vi "OpenTalonDrive (3).vi"   [LabVIEW 2016]
uses:
  <vilib>/Rock Robotics/WPI/ThirdParty/CanMotor/TalonSRX/WPI_CANTalonSRX_APIControlMode.ctl
  <vilib>/Rock Robotics/WPI/SafetyOutput/WPI_SafetyOutputConfigMenu.ctl
  <vilib>/Rock Robotics/WPI/ThirdParty/CanMotor/TalonSRX/WPI_CANTalonSRX_APIFeedbackSelect.ctl
types:
  T1 = typedef "WPI_CANTalonSRX_APIFeedbackSelect.ctl" = enum16{"Digital Quadrature Encoder", "Analog Potentiometer", "Analog Encoder", "Count on Quad-A (Rising-Edge)", "Count on Quad-A (Falling-Edge)", "CTR Magnetic Enc (Absolute)", "CTR Magnetic Enc (Relative)", "Pulse Width"}
  T2 = typedef "WPI_SafetyOutputConfigMenu.ctl" = enum16{"Enable", "Disable"}
  T3 = typedef "WPI_CANTalonSRX_APIControlMode.ctl" = enum8{"Percent VBus", "Speed", "Position", "Slave", "Unchanged / Invalid", "Voltage Compensation", "Current", "Motion Profile", "Motion Magic"}
  T4 = typedef "WPI_MotorControlDeviceRef.ctl" = cluster{"DeviceStatus":errorcluster, "Type":T5, "PWM":cluster{"PWM Channel":T6, "DeadBand":T7}, "CAN":cluster{"Device Number":u8, "SetOutput VI Ref":variant, "GetOutput VI Ref":variant, "Enable VI Ref":variant, "Disable VI Ref":variant, "Data":variant}, "Invert":bool}
  T5 = typedef "WPI_MotorControlType.ctl" = enum16{"PWM", "CAN"}
  T6 = typedef "FPGA_DIOPWMChannel.ctl" = enum8{"PWM 0", "PWM 1", "PWM 2", "PWM 3", "PWM 4", "PWM 5", "PWM 6", "PWM 7", "PWM 8", "PWM 9", "PWM MXP 0", "PWM MXP 1", "PWM MXP 2", "PWM MXP 3", "PWM MXP 4", "PWM MXP 5", "PWM MXP 6", "PWM MXP 7", "PWM MXP 8", "PWM MXP 9", "Invalid"}
  T7 = typedef "WPI_PWMDeadband.ctl" = cluster{"Name":string, "maxPositivePwm":i32, "minPositivePwm":i32, "centerPwm":i32, "maxNegativePwm":i32, "minNegativePwm":i32, "angularRange":u16}
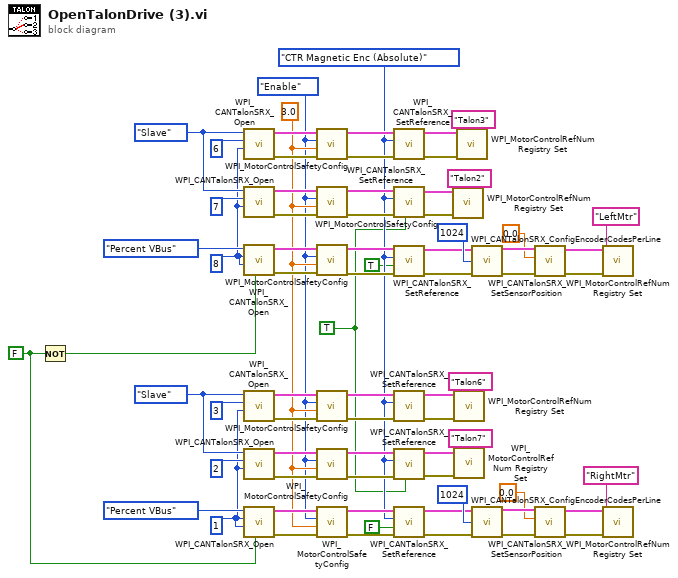
[diagram p0: block diagram]
diagram:
  w4 = FALSE
  w5 = TRUE
  w20 = WPI_CANTalonSRX_APIFeedbackSelect."CTR Magnetic Enc (Absolute)" ("Feedback Reference")
  w37 = WPI_SafetyOutputConfigMenu."Enable" ("mode")
  w7 = u8 1 ("Device Number")
  w55 = WPI_CANTalonSRX_APIControlMode."Slave" ("Control Mode")
  w38 = 3.0 ("timeout (s)")
  w6 = u8 8 ("Device Number")
  w72 = WPI_CANTalonSRX_APIControlMode."Slave" ("Control Mode")
  n1 = Not(x=w4) -> (.not. x?=w3:bool)
  n2 = call <vilib>:"WPI_CANTalonSRX_Open.vi"("Master Device Number"=w6, "Device Number"=u8 6, "Control Mode"=w72) -> ("error out"=w65:errorcluster, "CAN Talon SRX Ref"=w66:T4)  [unwired: 7 in]
  n3 = call <vilib>:"WPI_CANTalonSRX_Open.vi"("Master Device Number"=w6, "Device Number"=u8 7, "Control Mode"=w72) -> ("error out"=w63:errorcluster, "CAN Talon SRX Ref"=w64:T4)  [unwired: 7 in]
  n4 = call <vilib>:"WPI_CANTalonSRX_Open.vi"("Invert"=w3, "Master Device Number"=w6, "Device Number"=w6, "Control Mode"=WPI_CANTalonSRX_APIControlMode."Percent VBus") -> ("error out"=w67:errorcluster, "CAN Talon SRX Ref"=w68:T4)  [unwired: 6 in]
  n5 = call <vilib>:"WPI_CANTalonSRX_Open.vi"("Master Device Number"=w7, "Device Number"=u8 3, "Control Mode"=w55) -> ("error out"=w48:errorcluster, "CAN Talon SRX Ref"=w49:T4)  [unwired: 7 in]
  n6 = call <vilib>:"WPI_CANTalonSRX_Open.vi"("Master Device Number"=w7, "Device Number"=u8 2, "Control Mode"=w55) -> ("error out"=w46:errorcluster, "CAN Talon SRX Ref"=w47:T4)  [unwired: 7 in]
  n7 = call <vilib>:"WPI_CANTalonSRX_Open.vi"("Invert"=w4, "Master Device Number"=w7, "Device Number"=w7, "Control Mode"=WPI_CANTalonSRX_APIControlMode."Percent VBus") -> ("error out"=w50:errorcluster, "CAN Talon SRX Ref"=w51:T4)  [unwired: 6 in]
  n8 = call <vilib>:"WPI_MotorControlSafetyConfig.vi"("error in (no error)"=w65, "timeout (s)"=w38, "mode"=w37, "MotorControlDevRef"=w66) -> ("error out"=w35:errorcluster, "MotorControlDevRef"=w36:T4)  [unwired: 6 in]
  n9 = call <vilib>:"WPI_MotorControlSafetyConfig.vi"("error in (no error)"=w63, "timeout (s)"=w38, "mode"=w37, "MotorControlDevRef"=w64) -> ("error out"=w33:errorcluster, "MotorControlDevRef"=w34:T4)  [unwired: 6 in]
  n10 = call <vilib>:"WPI_MotorControlSafetyConfig.vi"("error in (no error)"=w67, "timeout (s)"=w38, "mode"=w37, "MotorControlDevRef"=w68) -> ("error out"=w23:errorcluster, "MotorControlDevRef"=w24:T4)  [unwired: 6 in]
  n11 = call <vilib>:"WPI_MotorControlSafetyConfig.vi"("error in (no error)"=w48, "timeout (s)"=w38, "mode"=w37, "MotorControlDevRef"=w49) -> ("error out"=w30:errorcluster, "MotorControlDevRef"=w29:T4)  [unwired: 6 in]
  n12 = call <vilib>:"WPI_MotorControlSafetyConfig.vi"("error in (no error)"=w46, "timeout (s)"=w38, "mode"=w37, "MotorControlDevRef"=w47) -> ("error out"=w32:errorcluster, "MotorControlDevRef"=w31:T4)  [unwired: 6 in]
  n13 = call <vilib>:"WPI_MotorControlSafetyConfig.vi"("error in (no error)"=w50, "timeout (s)"=w38, "mode"=w37, "MotorControlDevRef"=w51) -> ("error out"=w27:errorcluster, "MotorControlDevRef"=w28:T4)  [unwired: 6 in]
  n14 = call <vilib>:"WPI_CANTalonSRX_SetReference.vi"("error in (no error)"=w35, "Feedback Reference"=w20, "CAN Talon SRX Ref"=w36) -> ("error out"=w12:errorcluster, "CAN Talon SRX Ref"=w11:T4)  [unwired: 7 in]
  n15 = call <vilib>:"WPI_CANTalonSRX_SetReference.vi"("Reverse Closed-Loop Output"=w5, "error in (no error)"=w33, "Feedback Reference"=w20, "CAN Talon SRX Ref"=w34) -> ("error out"=w14:errorcluster, "CAN Talon SRX Ref"=w13:T4)  [unwired: 6 in]
  n16 = call <vilib>:"WPI_CANTalonSRX_SetReference.vi"("error in (no error)"=w23, "Reverse Feedback Sensor"=TRUE, "Feedback Reference"=w20, "CAN Talon SRX Ref"=w24) -> ("error out"=w21:errorcluster, "CAN Talon SRX Ref"=w22:T4)  [unwired: 6 in]
  n17 = call <vilib>:"WPI_CANTalonSRX_SetReference.vi"("error in (no error)"=w30, "Feedback Reference"=w20, "CAN Talon SRX Ref"=w29) -> ("error out"=w16:errorcluster, "CAN Talon SRX Ref"=w15:T4)  [unwired: 7 in]
  n18 = call <vilib>:"WPI_CANTalonSRX_SetReference.vi"("Reverse Closed-Loop Output"=w5, "error in (no error)"=w32, "Feedback Reference"=w20, "CAN Talon SRX Ref"=w31) -> ("error out"=w19:errorcluster, "CAN Talon SRX Ref"=w18:T4)  [unwired: 6 in]
  n19 = call <vilib>:"WPI_CANTalonSRX_SetReference.vi"("error in (no error)"=w27, "Reverse Feedback Sensor"=FALSE, "Feedback Reference"=w20, "CAN Talon SRX Ref"=w28) -> ("error out"=w25:errorcluster, "CAN Talon SRX Ref"=w26:T4)  [unwired: 6 in]
  n20 = call <vilib>:"WPI_MotorControlRefNum Registry Set.vi"("error in (no error)"=w14, "refnum name"="Talon2", "MotorControlDevRef"=w13) -> ()  [unwired: 7 in, 2 out]
  n21 = call <vilib>:"WPI_MotorControlRefNum Registry Set.vi"("error in (no error)"=w16, "refnum name"="Talon6", "MotorControlDevRef"=w15) -> ()  [unwired: 7 in, 2 out]
  n22 = call <vilib>:"WPI_MotorControlRefNum Registry Set.vi"("error in (no error)"=w19, "refnum name"="Talon7", "MotorControlDevRef"=w18) -> ()  [unwired: 7 in, 2 out]
  n23 = call <vilib>:"WPI_MotorControlRefNum Registry Set.vi"("error in (no error)"=w12, "refnum name"="Talon3", "MotorControlDevRef"=w11) -> ()  [unwired: 7 in, 2 out]
  n24 = call <vilib>:"WPI_CANTalonSRX_ConfigEncoderCodesPerLine.vi"("CAN Talon SRX Ref"=w22, "Number Encoder Lines\n(Counts Per Rotation)"=u32 1024 ("Number Encoder Lines\n(Counts Per Rotation)"), "error in (no error)"=w21) -> ("CAN Talon SRX Ref"=w60:T4, "error out"=w61:errorcluster)  [unwired: 11 in]
  n25 = call <vilib>:"WPI_CANTalonSRX_ConfigEncoderCodesPerLine.vi"("CAN Talon SRX Ref"=w26, "Number Encoder Lines\n(Counts Per Rotation)"=u32 1024 ("Number Encoder Lines\n(Counts Per Rotation)"), "error in (no error)"=w25) -> ("CAN Talon SRX Ref"=w43:T4, "error out"=w44:errorcluster)  [unwired: 11 in]
  n26 = call <vilib>:"WPI_CANTalonSRX_SetSensorPosition.vi"("error in (no error)"=w61, "New Sensor Position"=0.0, "CAN Talon SRX Ref"=w60) -> ("error out"=w58:errorcluster, "CAN Talon SRX Ref"=w57:T4)  [unwired: 7 in]
  n27 = call <vilib>:"WPI_CANTalonSRX_SetSensorPosition.vi"("error in (no error)"=w44, "New Sensor Position"=0.0, "CAN Talon SRX Ref"=w43) -> ("error out"=w41:errorcluster, "CAN Talon SRX Ref"=w40:T4)  [unwired: 7 in]
  n28 = call <vilib>:"WPI_MotorControlRefNum Registry Set.vi"("error in (no error)"=w58, "refnum name"="LeftMtr" ("Ref Name 1"), "MotorControlDevRef"=w57) -> ()  [unwired: 7 in, 2 out]
  n29 = call <vilib>:"WPI_MotorControlRefNum Registry Set.vi"("error in (no error)"=w41, "refnum name"="RightMtr" ("Ref Name 2"), "MotorControlDevRef"=w40) -> ()  [unwired: 7 in, 2 out]
